vi "TCP IP Server FGV.vi"() -> ()   [LabVIEW 2017]
panel:
  in  "Mode Selected":u16(ring) items=["Not Applicable", "Config Mode", "Manual Mode", "Auto Mode", "Simulation Mode", "Calibration Mode"]
  in  "Handshake":T1(ring)=enum."Machine Status"
  in  "Enum":T2(ring)
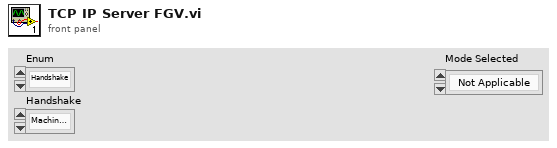
[diagram p1: front panel]
types:
  T1 = enum16{"Mode Selected", "Machine Status", "Alarm", "Software Error", "Emergency", "Safty ", "Spare 1", "Spare 2"}
  T2 = enum16{"Handshake", "Alarm", "Software Error", "Display Message", "Step Result", "Raw Data"}
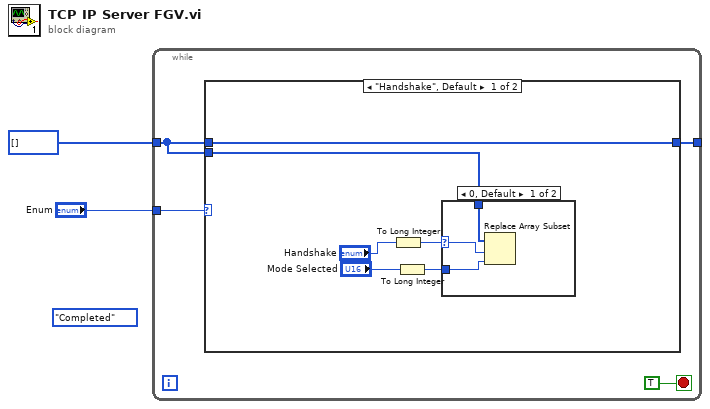
[diagram p0: block diagram]
diagram:
  (unwired) enum16{"Idle", "Running", "Completed"}."Completed"
  n1 = while {
    tunnel: "Enum" -> [w5]
    tunnel: i8[] [] -> [w3]
    tunnel: [w4] -> _
    stop <- TRUE stop-if-true
    n2 = case shown="\"Handshake\", Default" w5 {
      tunnel: w3 -> [w12 _]
      tunnel: [w12 _] -> w4
      tunnel: w3 -> [w11 _]
      frame "Handshake", Default {
        n3 = To Long Integer(number="Handshake") -> (32bit integer=w8:i32)
        n4 = To Long Integer(number="Mode Selected") -> (32bit integer=w7:i32)
        n5 = case shown="0, Default" w8 {
          selector: w8 -> [w14 _]
          tunnel: w11 -> [w15 _]
          tunnel: w7 -> [w13 _]
          frame 0, Default {
            n6 = Replace Array Subset(array=w15, new element=w13, index=w14) -> ()  [unwired: 1 out]
          }
          frame 1 {
          }
        }
      }
      frame "Alarm" {
      }
    }
  }
